vi "Enable-Disable.vi"(7 "Reference in":refnum<vi>, 8 "error in (no error)":errorcluster, 11 "E/D":T1(ring)=enum."Disabled and Grayed Out") -> (0 "error out":errorcluster)   [LabVIEW 2020]
doc: "This VI enable or disable controls/indicators."
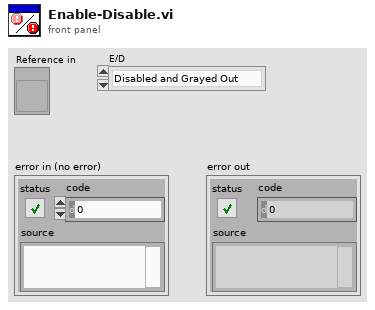
[diagram p1: front panel]
types:
  T1 = enum8{"Enabled", "Disabled", "Disabled and Grayed Out"}
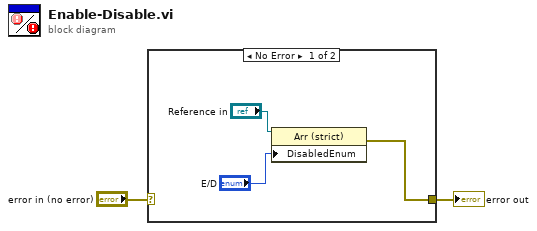
[diagram p0: block diagram]
diagram:
  n1 = case shown="No Error" "error in (no error)" {
    selector: "error in (no error)" -> [_ w6]
    tunnel: [w4 w6] -> w1
    frame No Error {
      n2 = property class="Arr (strict)"(reference="Reference in", "DisabledEnum"="E/D") -> (error out=w4:errorcluster)  [unwired: 1 in, 1 out]
    }
    frame Error {
    }
  }
  "error out" <- w1
